vi "AudioStreamer.CloseVI.vi"() -> (15 "error out":errorcluster)   [LabVIEW 2020]
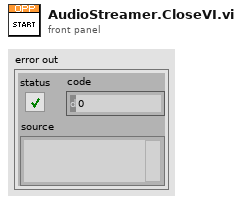
[diagram p1: front panel]
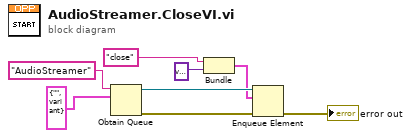
[diagram p0: block diagram]
diagram:
  n1 = Obtain Queue(name (unnamed)="AudioStreamer", element data type=cluster{string, variant} {"", variant}) -> (queue out=w5:refnum<queue>, error out=w6:errorcluster)  [unwired: 3 in, 1 out]
  n2 = Bundle("close", variant) -> (w2:cluster{string, variant})  [unwired: 1 in]
  n3 = Enqueue Element(queue=w5, element=w2, error in (no error)=w6) -> (error out=→"error out":errorcluster)  [unwired: 1 in, 2 out]
